vi "FormatTimeString.vi"(8 "error in (no error)":errorcluster, 10 "useUTC":bool, 11 "timestamp":timestamp) -> (0 "error out":errorcluster, 3 "timeString":string)   [LabVIEW 2026, in "Lumberjack.lvlib"]
doc: "Formats a LabVIEW timestamp as an ISO 8601 / RFC 3339 string with millisecond precision. Zone follows useUTC: 'Z' when UTC, otherwise a signed offset with a colon (+hh:mm). Shared by every layout's Format so all layouts render the same instant identically. Pure, no state."
uses:
  Lumberjack.lvlib
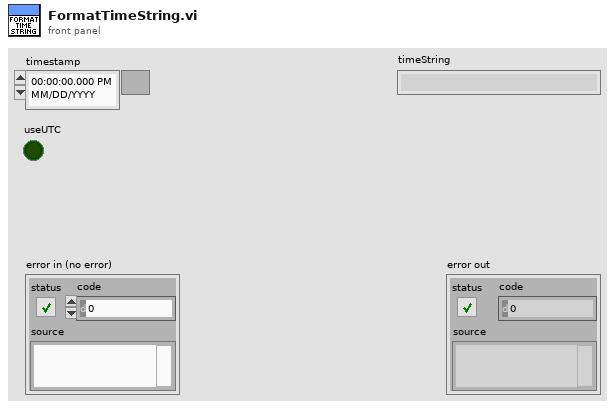
[diagram p1: front panel]
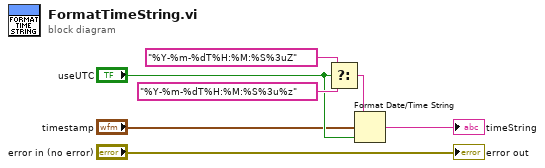
[diagram p0: block diagram]
diagram:
  n1 = Select(t="%Y-%m-%dT%H:%M:%S%3uZ" ("time format string (%c)"), s="useUTC", f="%Y-%m-%dT%H:%M:%S%3u%z" ("time format string (%c)")) -> (s? t:f=w7:string)
  n2 = Format Date/Time String(time format string (%c)=w7, seconds (now)="timestamp", UTC format="useUTC") -> (date/time string=→"timeString":string)
  "error out" <- "error in (no error)"
